vi "Test 1 Evaluate Card 1.vi"(8 "error in (no error)":errorcluster, 11 "Test Case In":refnum<class "Card evaluator Test.lvclass">) -> (0 "error out":errorcluster, 3 "Test Case Out":refnum<class "Card evaluator Test.lvclass">)   [LabVIEW 2020, in "Card evaluator Test.lvclass"]
uses:
  Card evaluator Test.lvclass
  Card evaluator Test.lvclass/Card evaluator Test.ctl
  4993e8ee-a06a-463a-9684-69129f64d5ce.vi
  Card/Card.lvclass
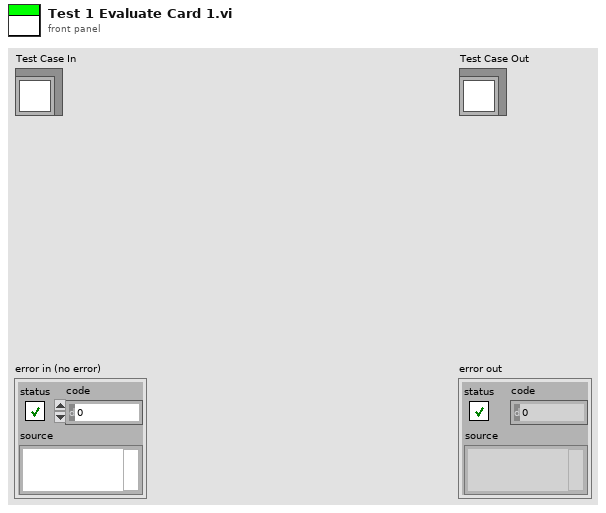
[diagram p1: front panel]
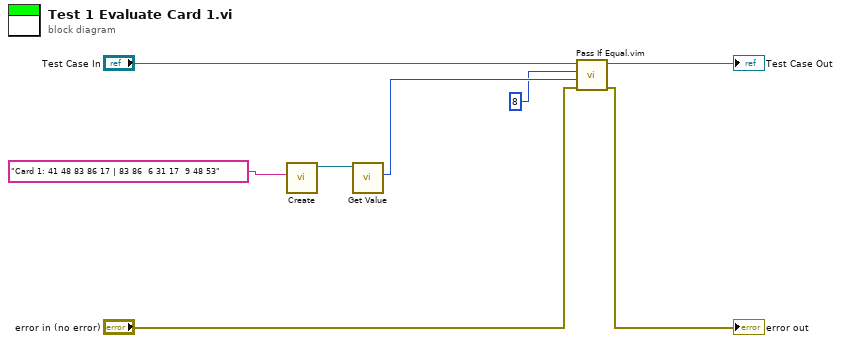
[diagram p0: block diagram]
diagram:
  n1 = call "Create.vi"("Card"="Card 1: 41 48 83 86 17 | 83 86  6 31 17  9 48 53") -> ("Card"=w3:refnum<class "Card.lvclass">)  [unwired: 9 in, 1 out]
  n2 = call-dynamic "Get Value.vi"("Card in"=w3) -> ("Value"=w2:i32)  [unwired: 8 in, 2 out]
  n3 = call "Pass If Equal.vim"("error in (no error)"="error in (no error)", "Actual"=w2, "Expected"=8 ("Value"), "LUnit Test Case In"="Test Case In") -> ("error out"=→"error out":errorcluster, "LUnit Test Case Out"=→"Test Case Out":refnum<class "Card evaluator Test.lvclass">)  [unwired: 6 in]
